vi "GenerateSyntheticData.vi"() -> ()   [LabVIEW 2013]
uses:
  BaesDataTypeDefinition.ctl
  <vilib>/Utility/file.llb/Write To Spreadsheet File (DBL).vi
  <vilib>/imath/engines/lvmath2/RunTimeEngine/NodeEndStatement/NIMS_NodeEndStatement_Output.vi
  <instcachedir>/0/NIMS_NodeEndStatement_Output_53EC0D466D134D7ABD903AC30B43404B.lvgen/NIMS_NodeEndStatement_Output_53EC0D466D134D7ABD903AC30B43404B_005.vi
  <vilib>/imath/engines/lvmath2/RunTimeEngine/ErrorHandling/NIMS_Finalize Error.vi
  <vilib>/gmath/statdist.llb/Normal Inverse CDF.vi
  <vilib>/gmath/NI_Gmath.lvlib
panel:
  out "appended array":dbl[](array[numeric])=[349.15, 349.61225, 350.0745, 350.53675, 350.999, 351.46125, 351.9235, 352.38575, 352.848, 353.31025, 353.7725, 354.23475, 354.697, 355.15925, 355.6215, 356.08375, 356.546, 357.00825, 357.4705, 357.93275, 358.395, 358.85725, 359.3195, 359.78175, 360.244, 360.70625, 361.1685, 361.63075, 362.093, 362.55525, 363.0175, 363.47975, 363.942, 364.40425, 364.8665, 365.32875, 365.791, 366.25325, 366.7155, 367.17775, 367.64, 368.10225, 368.5645, 369.02675, 369.489, 369.95125, 370.4135, 370.87575, 371.338, 371.80025, 372.2625, 372.72475, 373.187, 373.64925, 374.1115, 374.57375, 375.036, 375.49825, 375.9605, 376.42275, 376.885, 377.34725, 377.8095, 378.27175, 378.734, 379.19625, 379.6585, 380.12075, 380.583, 381.04525, 381.5075, 381.96975, 382.432, 382.89425, 383.3565, 383.81875, 384.281, 384.74325, 385.2055, 385.66775, 386.13, 386.59225, 387.0545, 387.51675, 387.979, 388.44125, 388.9035, 389.36575, 389.828, 390.29025, 390.7525, 391.21475, 391.677, 392.13925, 392.6015, 393.06375, 393.526, 393.98825, 394.4505, 394.91275, 395.375, 395.83725, 396.2995, 396.76175, 397.224, 397.68625, 398.1485, 398.61075, 399.073, 399.53525, 399.9975, 400.45975, 400.922, 401.38425, 401.8465, 402.30875, 402.771, 403.23325, 403.6955, 404.15775, 404.62, 405.08225, 405.5445, 406.00675, 406.469, 406.93125, 407.3935, 407.85575, 408.318, 408.78025, 409.2425, 409.70475, 410.167, 410.62925, 411.0915, 411.55375, 412.016, 412.47825, 412.9405, 413.40275, 413.865, 414.32725, 414.7895, 415.25175, 415.714, 416.17625, 416.6385, 417.10075, 417.563, 418.02525, 418.4875, 418.94975, 419.412, 419.87425, 420.3365]
  out "Expected Extinction Cross Section":sgl[][](array[numeric])=[[1.5946205e-09, 1.9495325e-09, 2.33351e-09, 2.7430718e-09, 3.1504757e-09, 3.5623626e-09, 3.998221e-09, 4.440756e-09], [1.6049403e-09, 1.9605007e-09, 2.3451892e-09, 2.7553189e-09, 3.161972e-09, 3.5725394e-09, 4.0074433e-09, 4.448538e-09], [1.6152926e-09, 1.9715136e-09, 2.3569386e-09, 2.767698e-09, 3.1736118e-09, 3.5828323e-09, 4.016789e-09, 4.4564503e-09], [1.6256803e-09, 1.982575e-09, 2.3687619e-09, 2.7802152e-09, 3.1854006e-09, 3.5932404e-09, 4.0262584e-09, 4.464491e-09], [1.6361074e-09, 1.9936892e-09, 2.380662e-09, 2.7928777e-09, 3.1973442e-09, 3.603768e-09, 4.0358503e-09, 4.472661e-09], [1.6465789e-09, 2.0048607e-09, 2.3926432e-09, 2.8056952e-09, 3.2094565e-09, 3.6144194e-09, 4.0455688e-09, 4.4809583e-09], [1.6570991e-09, 2.0160957e-09, 2.4047102e-09, 2.8186757e-09, 3.221743e-09, 3.6251995e-09, 4.0554173e-09, 4.4893884e-09], [1.6676729e-09, 2.0273994e-09, 2.4168694e-09, 2.8318308e-09, 3.2342196e-09, 3.6361156e-09, 4.065402e-09, 4.497954e-09], [1.6783054e-09, 2.0387785e-09, 2.4291262e-09, 2.8451723e-09, 3.246899e-09, 3.6471781e-09, 4.0755284e-09, 4.5066635e-09], [1.689001e-09, 2.0502395e-09, 2.4414868e-09, 2.858712e-09, 3.2597969e-09, 3.6583963e-09, 4.085806e-09, 4.515525e-09], [1.6997668e-09, 2.0617907e-09, 2.4539564e-09, 2.8724643e-09, 3.2729306e-09, 3.669782e-09, 4.0962447e-09, 4.52455e-09], [1.7106074e-09, 2.0734385e-09, 2.4665436e-09, 2.8864424e-09, 3.2863192e-09, 3.6813508e-09, 4.1068566e-09, 4.533751e-09], [1.7215274e-09, 2.0851925e-09, 2.479254e-09, 2.9006624e-09, 3.2999825e-09, 3.6931156e-09, 4.1176533e-09, 4.543145e-09], [1.7325316e-09, 2.0970594e-09, 2.4920943e-09, 2.9151401e-09, 3.3139447e-09, 3.705094e-09, 4.1286543e-09, 4.5527475e-09], [1.7436262e-09, 2.1090498e-09, 2.505072e-09, 2.929892e-09, 3.3282292e-09, 3.717305e-09, 4.1398724e-09, 4.562581e-09], [1.754815e-09, 2.121172e-09, 2.5181937e-09, 2.944936e-09, 3.3428638e-09, 3.7297694e-09, 4.1513273e-09, 4.5726685e-09], [1.7661018e-09, 2.1334354e-09, 2.5314653e-09, 2.9602896e-09, 3.3578764e-09, 3.7425085e-09, 4.1630384e-09, 4.583034e-09], [1.7774905e-09, 2.1458502e-09, 2.544894e-09, 2.9759704e-09, 3.3732965e-09, 3.7555488e-09, 4.17503e-09, 4.593709e-09], [1.7889845e-09, 2.1584252e-09, 2.5584848e-09, 2.9919975e-09, 3.3891592e-09, 3.768915e-09, 4.187325e-09, 4.6047246e-09], [1.8005847e-09, 2.1711728e-09, 2.5722433e-09, 3.008389e-09, 3.4054972e-09, 3.782637e-09, 4.199948e-09, 4.6161173e-09], [1.8122923e-09, 2.1841005e-09, 2.5861733e-09, 3.0251635e-09, 3.4223506e-09, 3.7967465e-09, 4.212929e-09, 4.627927e-09], [1.8241069e-09, 2.197221e-09, 2.6002789e-09, 3.0423386e-09, 3.439758e-09, 3.8112775e-09, 4.2262966e-09, 4.640197e-09], [1.8360258e-09, 2.2105435e-09, 2.6145632e-09, 3.0599312e-09, 3.4577614e-09, 3.826266e-09, 4.240083e-09, 4.6529762e-09], [1.8480469e-09, 2.2240794e-09, 2.6290277e-09, 3.0779583e-09, 3.4764063e-09, 3.8417527e-09, 4.2543227e-09, 4.6663176e-09], [1.8601631e-09, 2.2378384e-09, 2.6436724e-09, 3.0964324e-09, 3.495739e-09, 3.8577794e-09, 4.26905e-09, 4.680277e-09], [1.872366e-09, 2.2518323e-09, 2.6584968e-09, 3.1153673e-09, 3.5158094e-09, 3.8743924e-09, 4.2843022e-09, 4.6949187e-09], [1.884645e-09, 2.2660698e-09, 2.6734988e-09, 3.134772e-09, 3.5366685e-09, 3.8916417e-09, 4.300119e-09, 4.710311e-09], [1.896987e-09, 2.280562e-09, 2.6886737e-09, 3.1546534e-09, 3.5583698e-09, 3.9095807e-09, 4.3165405e-09, 4.726525e-09], [1.9093718e-09, 2.295318e-09, 2.704017e-09, 3.175013e-09, 3.5809686e-09, 3.928267e-09, 4.333608e-09, 4.7436415e-09], [1.9217787e-09, 2.3103466e-09, 2.7195215e-09, 3.1958483e-09, 3.6045211e-09, 3.9477603e-09, 4.3513624e-09, 4.761744e-09], [1.93418e-09, 2.3256561e-09, 2.73518e-09, 3.2171503e-09, 3.6290857e-09, 3.9681303e-09, 4.369848e-09, 4.7809228e-09], [1.9465445e-09, 2.3412534e-09, 2.750982e-09, 3.2389031e-09, 3.6547192e-09, 3.989446e-09, 4.3891033e-09, 4.801271e-09], [1.9588335e-09, 2.3571447e-09, 2.7669174e-09, 3.2610823e-09, 3.681478e-09, 4.011788e-09, 4.409171e-09, 4.8228874e-09], [1.9710018e-09, 2.373333e-09, 2.7829752e-09, 3.2836533e-09, 3.7094172e-09, 4.0352357e-09, 4.430089e-09, 4.8458766e-09], [1.9829982e-09, 2.3898208e-09, 2.7991451e-09, 3.3065737e-09, 3.73859e-09, 4.0598795e-09, 4.4518944e-09, 4.8703415e-09], [1.9947626e-09, 2.4066065e-09, 2.8154157e-09, 3.329784e-09, 3.7690437e-09, 4.0858166e-09, 4.474619e-09, 4.8963904e-09], [2.0062245e-09, 2.4236848e-09, 2.8317764e-09, 3.3532153e-09, 3.8008197e-09, 4.113147e-09, 4.498295e-09, 4.9241278e-09], [2.0173079e-09, 2.4410467e-09, 2.84822e-09, 3.3767813e-09, 3.8339505e-09, 4.1419836e-09, 4.5229465e-09, 4.953658e-09], [2.0279245e-09, 2.458677e-09, 2.864741e-09, 3.4003829e-09, 3.868458e-09, 4.17244e-09, 4.548594e-09, 4.9850764e-09], [2.0379753e-09, 2.4765554e-09, 2.8813358e-09, 3.423902e-09, 3.904347e-09, 4.204639e-09, 4.5752584e-09, 5.0184683e-09], [2.0473536e-09, 2.4946516e-09, 2.898006e-09, 3.4472065e-09, 3.9416084e-09, 4.238709e-09, 4.602959e-09, 5.0539035e-09], [2.0559394e-09, 2.5129272e-09, 2.914757e-09, 3.4701504e-09, 3.9802086e-09, 4.2747788e-09, 4.631712e-09, 5.0914344e-09], [2.0636062e-09, 2.5313314e-09, 2.9315983e-09, 3.4925722e-09, 4.020085e-09, 4.312983e-09, 4.661545e-09, 5.131076e-09], [2.0702164e-09, 2.5498015e-09, 2.9485434e-09, 3.5143006e-09, 4.061145e-09, 4.353448e-09, 4.6924957e-09, 5.172814e-09], [2.0756263e-09, 2.5682605e-09, 2.965609e-09, 3.5351617e-09, 4.1032564e-09, 4.396301e-09, 4.724618e-09, 5.2165805e-09], [2.0796898e-09, 2.586611e-09, 2.982816e-09, 3.554981e-09, 4.1462416e-09, 4.44165e-09, 4.7579944e-09, 5.26225e-09], [2.0822533e-09, 2.604738e-09, 3.0001834e-09, 3.5735923e-09, 4.18987e-09, 4.489595e-09, 4.7927395e-09, 5.3096243e-09], [2.0831703e-09, 2.6225049e-09, 3.01773e-09, 3.5908454e-09, 4.23385e-09, 4.5402033e-09, 4.8290065e-09, 5.3584226e-09], [2.0822988e-09, 2.6397489e-09, 3.0354708e-09, 3.6066186e-09, 4.2778265e-09, 4.593516e-09, 4.8669966e-09, 5.4082725e-09], [2.0795068e-09, 2.656282e-09, 3.0534109e-09, 3.6208248e-09, 4.321368e-09, 4.649529e-09, 4.9069544e-09, 5.4587095e-09], [2.0746822e-09, 2.6718892e-09, 3.0715457e-09, 3.6334193e-09, 4.3639665e-09, 4.708195e-09, 4.9491633e-09, 5.5091793e-09], [2.067733e-09, 2.6863243e-09, 3.0898522e-09, 3.6444097e-09, 4.405039e-09, 4.7694044e-09, 4.9939364e-09, 5.559071e-09], [2.0585986e-09, 2.6993143e-09, 3.1082878e-09, 3.6538585e-09, 4.443925e-09, 4.8329807e-09, 5.0415996e-09, 5.6077436e-09], [2.0472475e-09, 2.7105558e-09, 3.1267864e-09, 3.661875e-09, 4.4799044e-09, 4.8986704e-09, 5.092467e-09, 5.6545986e-09], [2.0336879e-09, 2.7197224e-09, 3.145249e-09, 3.6686216e-09, 4.512217e-09, 4.9661297e-09, 5.1468136e-09, 5.699157e-09], [2.017971e-09, 2.726465e-09, 3.1635448e-09, 3.6742922e-09, 4.5400874e-09, 5.0349143e-09, 5.2048525e-09, 5.7411444e-09], [2.0001831e-09, 2.7304243e-09, 3.181505e-09, 3.6791048e-09, 4.5627853e-09, 5.104465e-09, 5.2667004e-09, 5.7805796e-09], [1.980453e-09, 2.7312341e-09, 3.1989202e-09, 3.6832852e-09, 4.5796544e-09, 5.1741016e-09, 5.3323634e-09, 5.817828e-09], [1.958942e-09, 2.7285416e-09, 3.215537e-09, 3.6870438e-09, 4.590191e-09, 5.242999e-09, 5.401711e-09, 5.8536065e-09], [1.9358426e-09, 2.7220155e-09, 3.231058e-09, 3.6905647e-09, 4.5940913e-09, 5.3101736e-09, 5.4744684e-09, 5.8889427e-09], [1.9113682e-09, 2.7113698e-09, 3.2451415e-09, 3.6939802e-09, 4.5912967e-09, 5.3744915e-09, 5.5502145e-09, 5.925052e-09], [1.8857467e-09, 2.6963802e-09, 3.2574015e-09, 3.6973713e-09, 4.582024e-09, 5.434646e-09, 5.6283795e-09, 5.963201e-09], [1.8592061e-09, 2.6769025e-09, 3.2674154e-09, 3.700742e-09, 4.5667634e-09, 5.4891856e-09, 5.708252e-09, 6.0045355e-09], [1.8319747e-09, 2.6528906e-09, 3.2747265e-09, 3.7040269e-09, 4.546238e-09, 5.5365423e-09, 5.7889813e-09, 6.0499405e-09], [1.8042654e-09, 2.624407e-09, 3.2788554e-09, 3.707084e-09, 4.521347e-09, 5.5750906e-09, 5.8695937e-09, 6.0999295e-09], [1.7762711e-09, 2.5916322e-09, 3.279311e-09, 3.709694e-09, 4.493083e-09, 5.603251e-09, 5.948986e-09, 6.1545924e-09], [1.748163e-09, 2.5548588e-09, 3.275606e-09, 3.7115706e-09, 4.46244e-09, 5.6196026e-09, 6.025941e-09, 6.2135985e-09], [1.7200817e-09, 2.514486e-09, 3.2672767e-09, 3.7123622e-09, 4.430337e-09, 5.623037e-09, 6.0991163e-09, 6.2762338e-09], [1.6921434e-09, 2.470998e-09, 3.2539136e-09, 3.7116694e-09, 4.3975463e-09, 5.6129106e-09, 6.167058e-09, 6.341459e-09], [1.6644326e-09, 2.4249465e-09, 3.2351724e-09, 3.7090497e-09, 4.3646535e-09, 5.58915e-09, 6.2282033e-09, 6.4079977e-09], [1.6370073e-09, 2.3769144e-09, 3.2108098e-09, 3.704035e-09, 4.3320405e-09, 5.5523137e-09, 6.280908e-09, 6.474412e-09], [1.609903e-09, 2.3274949e-09, 3.1807064e-09, 3.6961518e-09, 4.2998827e-09, 5.5035767e-09, 6.3234795e-09, 6.53917e-09], [1.583133e-09, 2.2772588e-09, 3.1448812e-09, 3.6849306e-09, 4.268171e-09, 5.4446225e-09, 6.354258e-09, 6.6007027e-09], [1.5566949e-09, 2.2267375e-09, 3.1035126e-09, 3.6699301e-09, 4.2367407e-09, 5.377457e-09, 6.371703e-09, 6.65745e-09], [1.5305762e-09, 2.1764048e-09, 3.0569351e-09, 3.6507593e-09, 4.2053063e-09, 5.3042117e-09, 6.374524e-09, 6.7078894e-09], [1.5047519e-09, 2.12666e-09, 3.0056293e-09, 3.6270882e-09, 4.173498e-09, 5.2269336e-09, 6.3618115e-09, 6.7505614e-09], [1.4791994e-09, 2.0778368e-09, 2.9502127e-09, 3.5986767e-09, 4.1408974e-09, 5.147437e-09, 6.3331718e-09, 6.7840955e-09], [1.4538925e-09, 2.0301913e-09, 2.891396e-09, 3.5653855e-09, 4.107076e-09, 5.0671876e-09, 6.288814e-09, 6.8072326e-09], [1.4288131e-09, 1.983913e-09, 2.829959e-09, 3.5271934e-09, 4.0716137e-09, 4.987273e-09, 6.2295777e-09, 6.81886e-09], [1.4039466e-09, 1.9391346e-09, 2.7667042e-09, 3.4842036e-09, 4.0341344e-09, 4.90841e-09, 6.156892e-09, 6.8180595e-09], [1.3792927e-09, 1.895939e-09, 2.7024265e-09, 3.4366507e-09, 3.994326e-09, 4.8309916e-09, 6.0726433e-09, 6.804161e-09], [1.3548631e-09, 1.8543707e-09, 2.637875e-09, 3.3848944e-09, 3.9519583e-09, 4.755162e-09, 5.9790253e-09, 6.7767876e-09], [1.3306813e-09, 1.8144435e-09, 2.5737308e-09, 3.3294063e-09, 3.906886e-09, 4.6808775e-09, 5.878327e-09, 6.735921e-09], [1.3067861e-09, 1.7761527e-09, 2.5105893e-09, 3.270758e-09, 3.8590673e-09, 4.607982e-09, 5.7727676e-09, 6.6819177e-09], [1.2832301e-09, 1.7394796e-09, 2.4489497e-09, 3.209591e-09, 3.808567e-09, 4.5362647e-09, 5.6643503e-09, 6.6155263e-09], [1.2600763e-09, 1.7044e-09, 2.3892175e-09, 3.146593e-09, 3.7555394e-09, 4.4655026e-09, 5.55479e-09, 6.537846e-09], [1.2374023e-09, 1.6708889e-09, 2.331708e-09, 3.082471e-09, 3.7002414e-09, 4.395507e-09, 5.4454654e-09, 6.4502785e-09], [1.2152893e-09, 1.6389219e-09, 2.2766522e-09, 3.0179164e-09, 3.6430055e-09, 4.3261292e-09, 5.337431e-09, 6.3544396e-09], [1.1938278e-09, 1.6084818e-09, 2.2242164e-09, 2.9535905e-09, 3.5842338e-09, 4.257297e-09, 5.2314593e-09, 6.2520584e-09], [1.1731086e-09, 1.579558e-09, 2.1745015e-09, 2.890103e-09, 3.5243786e-09, 4.1890003e-09, 5.128093e-09, 6.144888e-09], [1.1532221e-09, 1.5521422e-09, 2.1275635e-09, 2.8279903e-09, 3.4639243e-09, 4.121298e-09, 5.0276867e-09, 6.0346097e-09], [1.1342559e-09, 1.5262352e-09, 2.0834217e-09, 2.7677207e-09, 3.4033703e-09, 4.0543093e-09, 4.9304707e-09, 5.9227667e-09], [1.1162921e-09, 1.5018414e-09, 2.042067e-09, 2.7096798e-09, 3.3432088e-09, 3.9882115e-09, 4.8365885e-09, 5.81074e-09], [1.0994033e-09, 1.4789674e-09, 2.0034705e-09, 2.6541787e-09, 3.283915e-09, 3.9232195e-09, 4.7461355e-09, 5.6997034e-09], [1.0836542e-09, 1.457624e-09, 1.9675883e-09, 2.6014602e-09, 3.2259322e-09, 3.859571e-09, 4.6591766e-09, 5.590642e-09], [1.0690959e-09, 1.4378181e-09, 1.9343656e-09, 2.5516949e-09, 3.1696585e-09, 3.7975267e-09, 4.5757638e-09, 5.4843445e-09], [1.055769e-09, 1.4195579e-09, 1.9037416e-09, 2.5049975e-09, 3.1154432e-09, 3.7373433e-09, 4.4959454e-09, 5.3814433e-09], [1.0437039e-09, 1.4028474e-09, 1.8756512e-09, 2.4614395e-09, 3.0635843e-09, 3.6792716e-09, 4.4197703e-09, 5.2824123e-09], [1.0329154e-09, 1.3876852e-09, 1.8500234e-09, 2.4210423e-09, 3.014322e-09, 3.6235452e-09, 4.34728e-09, 5.187615e-09], [1.0234095e-09, 1.3740653e-09, 1.8267882e-09, 2.3837945e-09, 2.9678453e-09, 3.5703676e-09, 4.2785206e-09, 5.0973026e-09], [1.0151815e-09, 1.3619758e-09, 1.8058709e-09, 2.3496616e-09, 2.9242906e-09, 3.5199215e-09, 4.2135313e-09, 5.011655e-09], [1.008216e-09, 1.3513972e-09, 1.7871951e-09, 2.3185809e-09, 2.8837532e-09, 3.472348e-09, 4.152336e-09, 4.930778e-09], [1.0024898e-09, 1.3423046e-09, 1.7706845e-09, 2.2904723e-09, 2.84628e-09, 3.4277576e-09, 4.094946e-09, 4.854718e-09], [9.979723e-10, 1.334668e-09, 1.7562587e-09, 2.2652464e-09, 2.8118798e-09, 3.3862284e-09, 4.0413664e-09, 4.7834887e-09], [9.946264e-10, 1.3284482e-09, 1.7438383e-09, 2.242801e-09, 2.780537e-09, 3.3478007e-09, 3.991576e-09, 4.7170525e-09], [9.924112e-10, 1.3236047e-09, 1.7333404e-09, 2.223026e-09, 2.7522065e-09, 3.3124872e-09, 3.9455363e-09, 4.6553508e-09], [9.912796e-10, 1.3200885e-09, 1.7246821e-09, 2.2058042e-09, 2.7268163e-09, 3.280272e-09, 3.9031973e-09, 4.5982915e-09], [9.911835e-10, 1.3178502e-09, 1.7177795e-09, 2.19102e-09, 2.704282e-09, 3.2511158e-09, 3.864483e-09, 4.5457687e-09], [9.92071e-10, 1.3168341e-09, 1.7125473e-09, 2.1785518e-09, 2.6845028e-09, 3.224951e-09, 3.8293066e-09, 4.497648e-09], [9.938899e-10, 1.3169841e-09, 1.7088997e-09, 2.1682776e-09, 2.6673692e-09, 3.2017005e-09, 3.7975654e-09, 4.4537853e-09], [9.965877e-10, 1.3182417e-09, 1.7067537e-09, 2.160077e-09, 2.6527631e-09, 3.1812688e-09, 3.7691463e-09, 4.4140243e-09], [1.00011e-09, 1.3205468e-09, 1.7060233e-09, 2.153832e-09, 2.6405598e-09, 3.1635459e-09, 3.7439194e-09, 4.378198e-09], [1.0044044e-09, 1.3238397e-09, 1.7066262e-09, 2.1494226e-09, 2.630633e-09, 3.1484164e-09, 3.7217542e-09, 4.346131e-09], [1.009419e-09, 1.3280599e-09, 1.70848e-09, 2.1467368e-09, 2.6228533e-09, 3.135758e-09, 3.7025074e-09, 4.317641e-09], [1.0151027e-09, 1.3331485e-09, 1.7115042e-09, 2.1456603e-09, 2.6170957e-09, 3.125443e-09, 3.6860381e-09, 4.29255e-09], [1.0214066e-09, 1.3390462e-09, 1.7156224e-09, 2.1460853e-09, 2.6132334e-09, 3.117341e-09, 3.6721952e-09, 4.2706705e-09], [1.0282825e-09, 1.3456972e-09, 1.7207566e-09, 2.147909e-09, 2.6111422e-09, 3.1113225e-09, 3.6608347e-09, 4.251821e-09], [1.0356842e-09, 1.3530458e-09, 1.7268356e-09, 2.1510296e-09, 2.6107034e-09, 3.1072613e-09, 3.6518062e-09, 4.235821e-09], [1.0435682e-09, 1.3610375e-09, 1.733788e-09, 2.1553506e-09, 2.6117986e-09, 3.1050282e-09, 3.644964e-09, 4.2224904e-09], [1.0518925e-09, 1.3696219e-09, 1.7415474e-09, 2.1607824e-09, 2.614319e-09, 3.1045002e-09, 3.6401682e-09, 4.211656e-09], [1.0606167e-09, 1.3787494e-09, 1.7500492e-09, 2.1672366e-09, 2.6181548e-09, 3.1055583e-09, 3.6372794e-09, 4.203151e-09], [1.0697032e-09, 1.3883736e-09, 1.7592324e-09, 2.1746307e-09, 2.6232068e-09, 3.1080853e-09, 3.6361638e-09, 4.1968127e-09], [1.0791156e-09, 1.3984488e-09, 1.769038e-09, 2.182887e-09, 2.629376e-09, 3.1119725e-09, 3.6366925e-09, 4.1924846e-09], [1.0888213e-09, 1.4089347e-09, 1.7794134e-09, 2.1919324e-09, 2.636572e-09, 3.1171143e-09, 3.6387449e-09, 4.19002e-09], [1.0987877e-09, 1.4197903e-09, 1.7903059e-09, 2.2016982e-09, 2.6447098e-09, 3.123412e-09, 3.6422036e-09, 4.189275e-09], [1.1089847e-09, 1.4309789e-09, 1.8016675e-09, 2.2121183e-09, 2.6537057e-09, 3.1307688e-09, 3.6469563e-09, 4.1901185e-09], [1.1193847e-09, 1.4424654e-09, 1.8134532e-09, 2.2231337e-09, 2.6634868e-09, 3.139099e-09, 3.652899e-09, 4.1924224e-09], [1.1299615e-09, 1.4542164e-09, 1.8256199e-09, 2.2346884e-09, 2.6739804e-09, 3.1483176e-09, 3.6599355e-09, 4.1960675e-09], [1.1406907e-09, 1.4662026e-09, 1.8381301e-09, 2.2467295e-09, 2.6851221e-09, 3.1583476e-09, 3.6679728e-09, 4.200943e-09], [1.1515502e-09, 1.4783951e-09, 1.8509454e-09, 2.2592066e-09, 2.6968479e-09, 3.1691147e-09, 3.6769239e-09, 4.2069463e-09], [1.1625179e-09, 1.4907676e-09, 1.864034e-09, 2.2720783e-09, 2.7091036e-09, 3.1805536e-09, 3.6867103e-09, 4.213977e-09], [1.1735746e-09, 1.5032962e-09, 1.8773627e-09, 2.2853004e-09, 2.721835e-09, 3.1926009e-09, 3.6972574e-09, 4.2219472e-09], [1.1847021e-09, 1.5159578e-09, 1.890905e-09, 2.2988365e-09, 2.734994e-09, 3.2051994e-09, 3.708495e-09, 4.2307717e-09], [1.1958843e-09, 1.5287333e-09, 1.9046345e-09, 2.3126505e-09, 2.7485372e-09, 3.2182959e-09, 3.720362e-09, 4.2403747e-09], [1.2071051e-09, 1.5416021e-09, 1.9185262e-09, 2.3267115e-09, 2.7624236e-09, 3.2318415e-09, 3.732799e-09, 4.2506842e-09], [1.2183506e-09, 1.5545488e-09, 1.93256e-09, 2.34099e-09, 2.7766145e-09, 3.2457912e-09, 3.745754e-09, 4.261634e-09], [1.229608e-09, 1.5675566e-09, 1.946715e-09, 2.3554605e-09, 2.7910767e-09, 3.260106e-09, 3.759176e-09, 4.2731636e-09], [1.2408649e-09, 1.5806123e-09, 1.9609738e-09, 2.3700975e-09, 2.805781e-09, 3.2747476e-09, 3.773023e-09, 4.2852206e-09], [1.2521105e-09, 1.5937023e-09, 1.975322e-09, 2.38488e-09, 2.8206972e-09, 3.289683e-09, 3.7872536e-09, 4.2977524e-09], [1.2633349e-09, 1.6068156e-09, 1.9897437e-09, 2.3997908e-09, 2.8358025e-09, 3.3048817e-09, 3.8018313e-09, 4.3107153e-09], [1.2745286e-09, 1.6199416e-09, 2.0042281e-09, 2.4148112e-09, 2.8510734e-09, 3.3203182e-09, 3.8167247e-09, 4.3240673e-09], [1.2856841e-09, 1.6330716e-09, 2.0187643e-09, 2.4299267e-09, 2.8664893e-09, 3.3359666e-09, 3.831906e-09, 4.3377724e-09], [1.2967935e-09, 1.6461976e-09, 2.033342e-09, 2.4451237e-09, 2.8820337e-09, 3.3518088e-09, 3.8473473e-09, 4.351797e-09], [1.3078493e-09, 1.6593131e-09, 2.0479543e-09, 2.4603928e-09, 2.8976912e-09, 3.3678236e-09, 3.863028e-09, 4.3661137e-09], [1.3188468e-09, 1.6724104e-09, 2.0625943e-09, 2.4757225e-09, 2.9134481e-09, 3.3839966e-09, 3.8789287e-09, 4.3806954e-09], [1.3297794e-09, 1.6854865e-09, 2.077258e-09, 2.4911067e-09, 2.9292946e-09, 3.4003145e-09, 3.895034e-09, 4.3955217e-09], [1.3406419e-09, 1.6985352e-09, 2.0919395e-09, 2.5065379e-09, 2.9452183e-09, 3.4167646e-09, 3.911329e-09, 4.4105706e-09], [1.3514307e-09, 1.7115538e-09, 2.1066373e-09, 2.522012e-09, 2.9612146e-09, 3.433339e-09, 3.9278034e-09, 4.425829e-09], [1.3621411e-09, 1.724539e-09, 2.121349e-09, 2.5375244e-09, 2.9772744e-09, 3.45003e-09, 3.9444488e-09, 4.441283e-09], [1.3727685e-09, 1.7374882e-09, 2.136074e-09, 2.553075e-09, 2.9933944e-09, 3.4668326e-09, 3.961259e-09, 4.4569206e-09], [1.383311e-09, 1.7503997e-09, 2.1508122e-09, 2.5686613e-09, 3.0095733e-09, 3.4837435e-09, 3.97823e-09, 4.472738e-09], [1.3937637e-09, 1.7632715e-09, 2.1655637e-09, 2.5842832e-09, 3.0258054e-09, 3.5007597e-09, 3.9953596e-09, 4.4887254e-09], [1.4041253e-09, 1.7761036e-09, 2.180332e-09, 2.5999425e-09, 3.0420926e-09, 3.5178802e-09, 4.0126493e-09, 4.504883e-09], [1.4143915e-09, 1.7888948e-09, 2.195118e-09, 2.6156428e-09, 3.0584342e-09, 3.5351082e-09, 4.0301007e-09, 4.5212083e-09], [1.4245604e-09, 1.8016444e-09, 2.209925e-09, 2.6313853e-09, 3.0748322e-09, 3.5524452e-09, 4.0477177e-09, 4.5377044e-09]]
  out "Concentration":dbl[][](array[numeric])
  out "Sizes":dbl[](array[numeric])
  out "GeometricCrossSection":dbl[](array[numeric])=[5.939573610693203e-10, 7.068583470577035e-10, 8.295768100885549e-10, 9.621127501618742e-10, 1.1044661672776617e-09, 1.2566370614359174e-09, 1.418625432636641e-09, 1.590431280879833e-09]
  out "Number ofSizes":dbl=8.0
  out "Size parameters":dbl[](array[numeric])=[2.0553484642356614, 2.2421983246207216, 2.4290481850057817, 2.615898045390842, 2.802747905775902, 2.989597766160962, 3.176447626546022, 3.3632974869310823]
  out "Numeric":i32=154
  out "size(s)":i32=155
  in  "Population Size":i32=1
  in  "Extinction ExtinctionUncertainity Size parameter and Number ofS sizes":T1={"Extinction"=[], "Extinction Uncertainty"=[], "Size parameters"=[], "Number ofSizes"=0.0, "GeometricCrossSection"=[], "Wave Length"=0.0, "SMPS Sizes"=[], "Concentration"=[], "Double Charge Correction"=FALSE, "Extincation Factor"=1.0, "Diameter Factor"=1.0, "Diameter Offset"=0.0, "Extinction Factor Flag"=FALSE, "Diameter Factor Flag"=FALSE, "Diameter Offset Flag"=FALSE, "Sizes"=[], "ExtinctionOrAbsorptionOrScattering"=0} {"ExtinctionOrAbsorptionOrScattering" scale=0.0..2.0}
  in  "Extinction File 2":path=path "Z:/Dropbox/Lior Segev/Lior Segev Projects/RI retrieval in Labview/Data/Nir/PAS fake data/GeneratedPASAmplitudes.txt"
  out "Double Charge correction Initiated":bool=TRUE
  in  "Particle Concentration File":path=path "Z:/Dropbox/Lior Segev/Lior Segev Projects/RI retrieval in Labview/Data/Nir/PAS fake data/MCD PAS fake absorption data.txt"
  in  "Extinction File":path=path "Z:/Dropbox/Lior Segev/Lior Segev Projects/RI retrieval in Labview/Data/Nir/PAS fake data/PAS fake absorption data.txt"
  out "Number of Different Wavelengths":i32=155
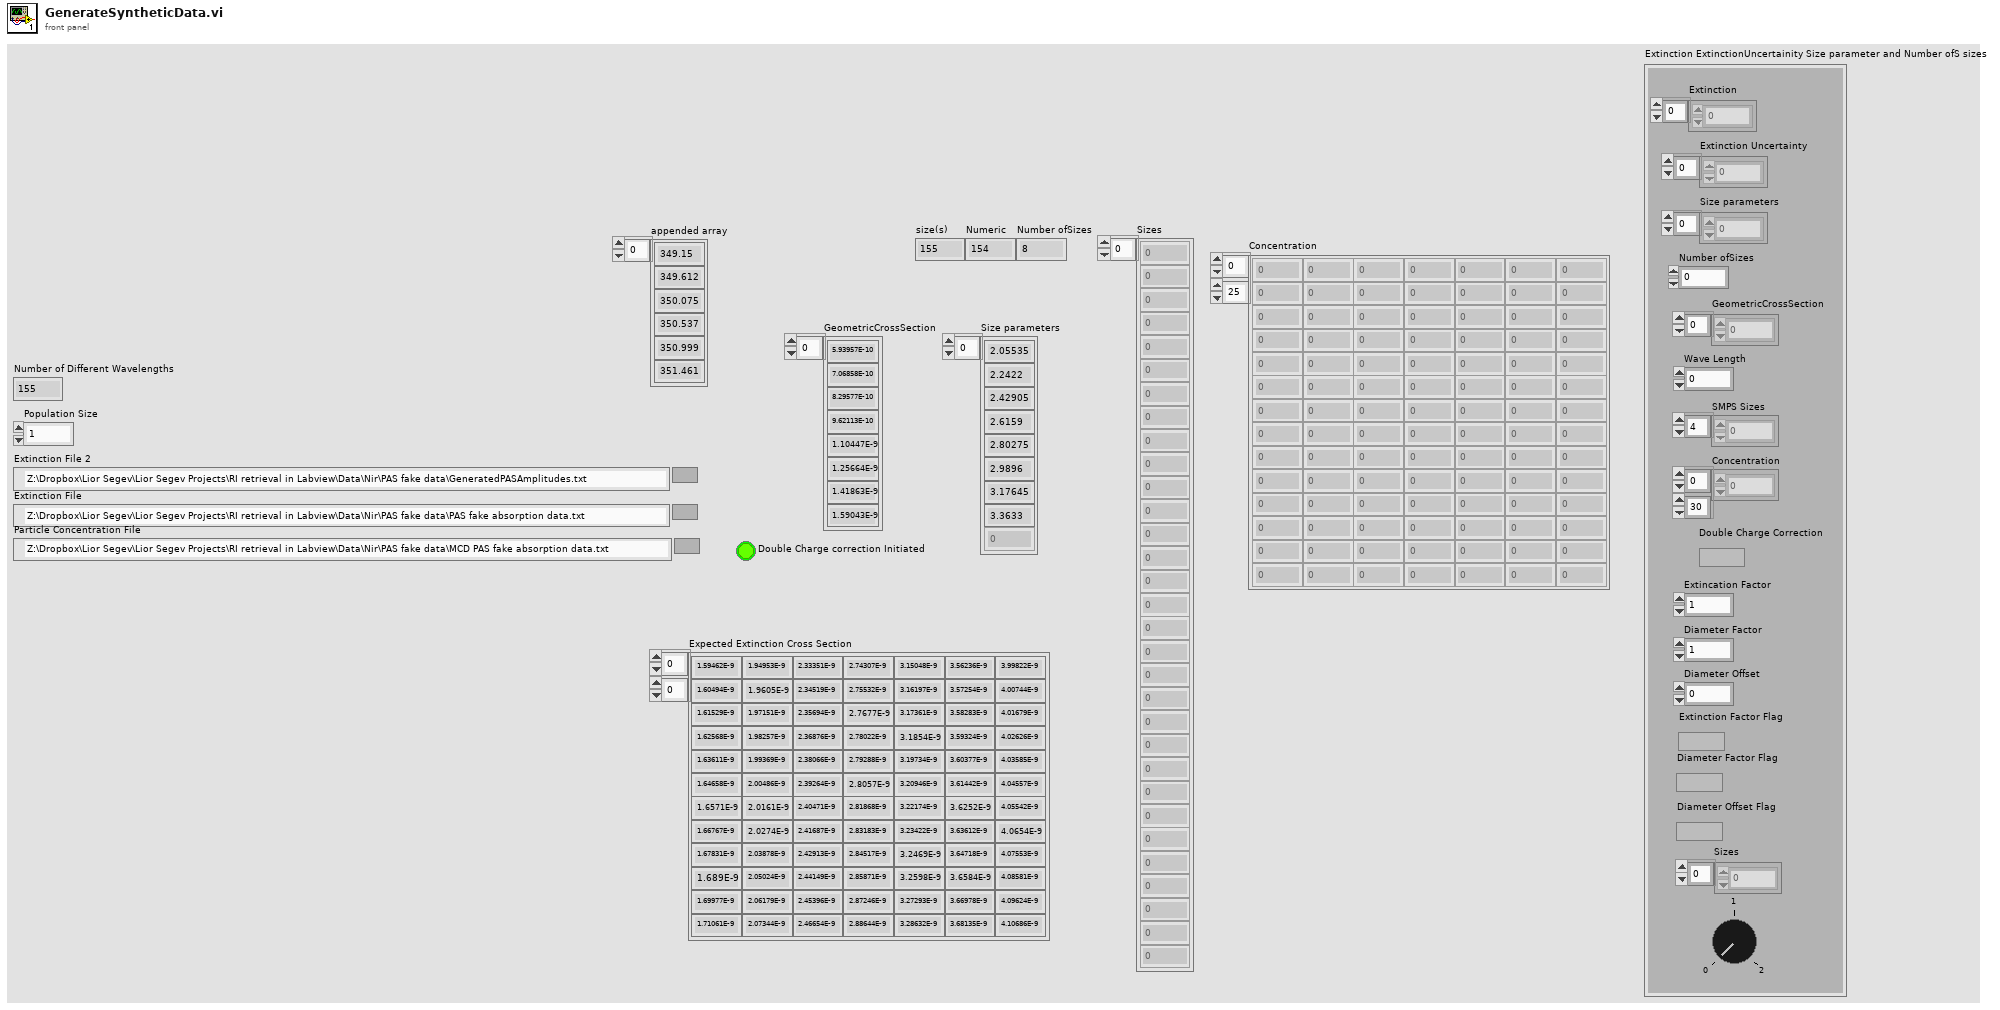
[diagram p1: front panel]
types:
  T1 = typedef "BaesDataTypeDefinition.ctl" = cluster{"Extinction":dbl[], "Extinction Uncertainty":dbl[], "Size parameters":dbl[], "Number ofSizes":dbl, "GeometricCrossSection":dbl[], "Wave Length":dbl, "SMPS Sizes":dbl[], "Concentration":dbl[][], "Double Charge Correction":bool, "Extincation Factor":dbl, "Diameter Factor":dbl, "Diameter Offset":dbl, "Extinction Factor Flag":bool, "Diameter Factor Flag":bool, "Diameter Offset Flag":bool, "Sizes":dbl[], "ExtinctionOrAbsorptionOrScattering":i8}
  T2 = typedef "ReadBaesDataTypeDefinition.ctl" = cluster{"Extinction":dbl[][], "Extinction Uncertainty":dbl[][], "Size parameters":dbl[][], "Number ofSizes":dbl, "GeometricCrossSection":dbl[], "WaveLength":dbl[], "Sizes":dbl[], "Concentration (#/cc)":dbl[]}
  T3 = typedef "ParticleDistributionData.ctl" = cluster{"SMPS Sizes":dbl[], "Concentration":dbl[][], "Double Charge Correction Flag":bool}
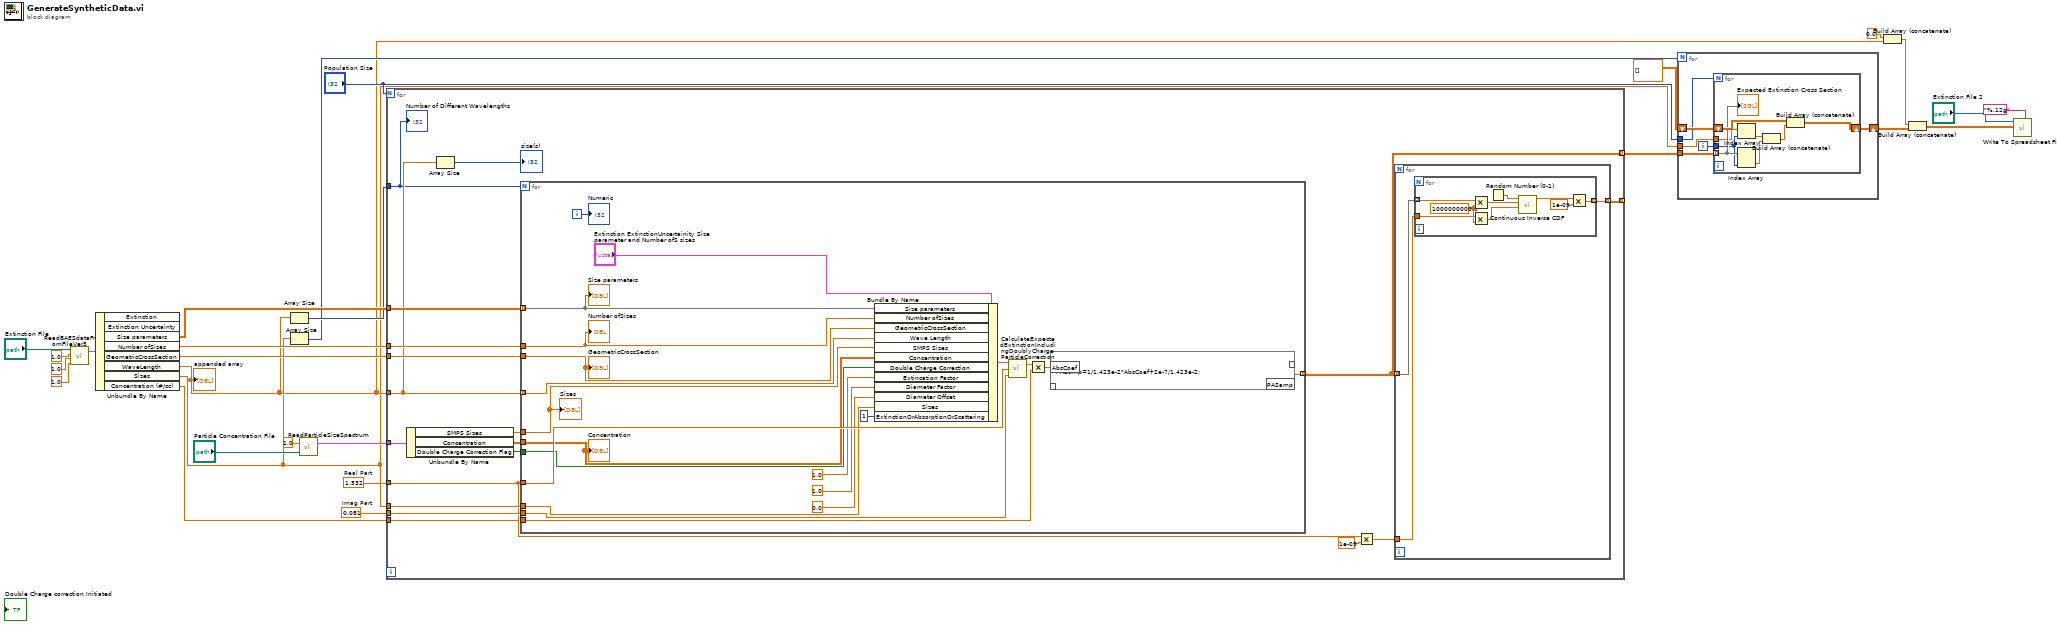
[diagram p0: block diagram]
diagram:
  w2 = 0.081  # Imag Part
  w3 = 1.532  # Real Part
  n1 = call "ReadBAESdataFromFileVer3.vi"("Factor Size Parameter"=1.0, "Factor Extinction"=1.0, "Factor Ext Uncertainty"=1.0, "file path"="Extinction File") -> ("Extinction ExtinctionUncertainity Size parameter and Number ofS sizes"=w23:T2)  [unwired: 1 out]
  n2 = Unbundle By Name(w23) -> ("Size parameters"=w21:dbl[][], "Number ofSizes"=w20:dbl, "GeometricCrossSection"=w19:dbl[], "WaveLength"=w11:dbl[], "Sizes"=w5:dbl[], "Concentration (#/cc)"=w1:dbl[])  [unwired: 2 out]
  "appended array" <- w11
  n3 = Array Size(array=w11) -> (size(s)=w18:i32)
  n4 = Array Size(array=w5) -> (size(s)=w15:i32)
  n5 = call "ReadParticleSizeSpectrum.vi"("file path"="Particle Concentration File", "Factor Size paramter"=1.0) -> ("Particle Distribution Data"=w22:T3)  [unwired: 1 out]
  n6 = for {
    N: "Population Size" -> [_]
    tunnel: w22 -> [w45]
    tunnel: w21 -> [w44]
    tunnel: w20 -> [w43]
    tunnel: w19 -> [w42]
    tunnel: w11 -> [w37]
    tunnel: w18 -> [w36]
    tunnel: w3 -> [w29]
    tunnel: w2 -> [w34]
    tunnel: [w35] -> _ mode=indexing
    tunnel: w5 -> [w31]
    tunnel: [w30] -> w4 mode=indexing
    tunnel: w1 -> [w28]
    n7 = Unbundle By Name(w45) -> ("SMPS Sizes"=w39:dbl[], "Concentration"=w41:dbl[][], "Double Charge Correction Flag"=w40:bool)
    n8 = Array Size(array=w37) -> (size(s)=→"size(s)":i32)
    n9 = for {
      N: w36 -> [_]
      tunnel: w29 -> [w78]
      tunnel: w34 -> [w63]
      tunnel: [w58] -> w30 mode=indexing
      tunnel: w44 -> [w75] mode=indexing
      tunnel: w43 -> [w74]
      tunnel: w42 -> [w73]
      tunnel: w37 -> [w72] mode=indexing
      tunnel: w39 -> [w71]
      tunnel: w41 -> [w70]
      tunnel: w40 -> [w69]
      tunnel: w31 -> [w65]
      tunnel: w28 -> [w60]
      i -> [w68]
      n10 = Bundle By Name(cluster="Extinction ExtinctionUncertainity Size parameter and Number ofS sizes", "Size parameters"=w75, "Number ofSizes"=w74, "GeometricCrossSection"=w73, "Wave Length"=w72, "SMPS Sizes"=w71, "Concentration"=w70, "Double Charge Correction"=w69, "Extincation Factor"=1.0, "Diameter Factor"=1.0, "Diameter Offset"=0.0, "Sizes"=w65, "ExtinctionOrAbsorptionOrScattering"=i8 1) -> (w76:T1)
      n11 = call "CalculateExpectedExtinctionIncludingDoublyChargeParticleCorrection.vi"("refractive index, imaginary"=w63, "refractive index, real"=w78, "Extinction ExtinctionUncertainity Size parameter and Number ofS sizes"=w76) -> ("Expected Extinction Cross Section"=w61:sgl[])  [unwired: 1 out]
      n12 = Multiply(x=w61, y=w60) -> (x*y=w59:dbl[])
      n13 = mathscript code="PASamp=1/1.423e-2*AbsCoef+2e-7/1.423e-2;"("AbsCoef"=w59) -> ("PASamp"=w58:dbl[])  [unwired: 1 in, 1 out]
      "Numeric" <- w68
      "Size parameters" <- w75
      "Number ofSizes" <- w74
      "GeometricCrossSection" <- w73
      "Sizes" <- w71
      "Concentration" <- w70
    }
    n14 = Multiply(x=w29, y=1e-09) -> (x*y=w33:dbl)
    n15 = for {
      tunnel: w30 -> [w48] mode=indexing
      tunnel: w33 -> [w47]
      tunnel: [w46] -> w35 mode=indexing
      n16 = for {
        tunnel: w48 -> [w56] mode=indexing
        tunnel: w47 -> [w54]
        tunnel: [w49] -> w46 mode=indexing
        w53 = 1000000000.0 ("y")
        n17 = Multiply(x=w56, y=w53) -> (x*y=w55:dbl)
        n18 = Multiply(x=w54, y=w53) -> (x*y=w52:dbl)
        n19 = Random Number (0-1)() -> (number: 0 to 1=w57:dbl)
        n20 = call-poly <vilib>:"Continuous Inverse CDF.vi"("std"=w52, "mean"=w55, "cdf(x)"=w57) -> ("x"=w51:dbl)  [unwired: 7 in, 1 out]
        n21 = Multiply(x=w51, y=1e-09) -> (x*y=w49:dbl)
      }
    }
    "Number of Different Wavelengths" <- w36
  }
  n22 = for {
    N: w15 -> [_]
    tunnel: w4 -> [w107]
    tunnel: "Population Size" -> [w105]
    tunnel: w5 -> [w104]
    shift-right: [w103] -> w13
    shift-left: sgl[][] [] ("Expected Extinction Cross Section") -> [w106]
    i -> [w102]
    n23 = for {
      N: w105 -> [_]
      tunnel: w107 -> [w113] mode=indexing
      shift-right: [w114] -> w103
      shift-left: w106 -> [w115]
      tunnel: w104 -> [w112]
      tunnel: w102 -> [w108]
      n24 = Index Array(array=w112, index=w108) -> (element=w111:dbl)
      n25 = Index Array(array=w113, index (col)=w108) -> (element=w110:dbl[])  [unwired: 1 in]
      n26 = Build Array (concatenate)(w111, w110) -> (w109:dbl[])
      n27 = Build Array (concatenate)(w115, w109) -> (w114:dbl[][])
      "Expected Extinction Cross Section" <- w113
    }
  }
  n28 = Build Array (concatenate)(0.0 ("element"), w11) -> (w10:dbl[])
  n29 = Build Array (concatenate)(w10, w13) -> (w12:dbl[][])
  n30 = call-poly <vilib>:"Write To Spreadsheet File.vi"("format (%.3f)"="%.12g", "2D data"=w12, "file path (dialog if empty)"="Extinction File 2") -> ()  [unwired: 5 in, 1 out]
